vi "serialization tests.vi"() -> (0 "error out":errorcluster, 2 "success?":bool)   [LabVIEW 2013, in "shared memory tests.lvlib"]
doc: "Tests the 'To String' and 'From String' methods of the Module's configuration class and ensures they are compatible."
uses:
  shared memory tests.lvlib
  module/configuration/shared memory configuration.lvclass
  module/configuration/shared memory configuration.lvclass/shared memory configuration.ctl
  <vilib>/NI/Tag Bus Module Framework/channel/TBM channel.lvclass
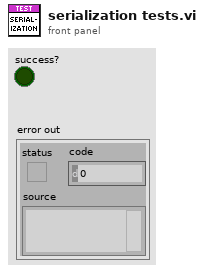
[diagram p1: front panel]
types:
  T1 = typedef "shared memory configuration.lvclass/Line.ctl" = cluster{"channel":refnum<class "TBM channel.lvclass">}
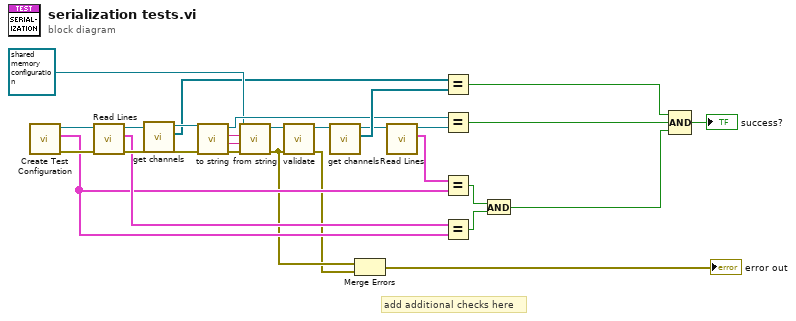
[diagram p0: block diagram]
diagram:
  # "add additional checks here"
  n1 = call "Create Test Configuration.vi"() -> ("error out"=w15:errorcluster, "Line Array"=w10:T1[], "Module Configuration"=w13:refnum<class "shared memory configuration.lvclass">)  [unwired: 6 in, 3 out]
  n2 = call "Read Lines.vi"("error in (no error)"=w15, "shared memory configuration in"=w13) -> ("error out"=w14:errorcluster, "Lines"=w11:T1[], "shared memory configuration out"=w12:refnum<class "shared memory configuration.lvclass">)  [unwired: 7 in]
  n3 = call-dynamic "get channels.vi"("shared memory configuration in"=w12) -> ("channels"=w19:refnum<class "TBM channel.lvclass">[], "shared memory configuration out"=w20:refnum<class "shared memory configuration.lvclass">)  [unwired: 9 in]
  n4 = call-dynamic "to string.vi"("error in"=w14, "shared memory configuration in"=w20) -> ("error out"=w28:errorcluster, "data"=w27:string, "version"=w26:string, "shared memory configuration out"=w22:refnum<class "shared memory configuration.lvclass">)  [unwired: 6 in]
  n5 = call-dynamic "from string.vi"("error in"=w28, "data"=w27, "version"=w26, "shared memory configuration in"=refnum<class "shared memory configuration.lvclass"> refnum ("tag bus configurable plugin module configuration")) -> ("error out"=w7:errorcluster, "shared memory configuration out"=w25:refnum<class "shared memory configuration.lvclass">)  [unwired: 6 in]
  n6 = call-dynamic "validate.vi"("error in"=w7, "shared memory configuration in"=w25) -> ("error out"=w6:errorcluster, "shared memory configuration out"=w24:refnum<class "shared memory configuration.lvclass">)  [unwired: 8 in]
  n7 = call-dynamic "get channels.vi"("shared memory configuration in"=w24) -> ("channels"=w23:refnum<class "TBM channel.lvclass">[], "shared memory configuration out"=w18:refnum<class "shared memory configuration.lvclass">)  [unwired: 9 in]
  n8 = Merge Errors(w7, w6) -> (→"error out":errorcluster)
  n9 = call "Read Lines.vi"("shared memory configuration in"=w18) -> ("Lines"=w16:T1[], "shared memory configuration out"=w17:refnum<class "shared memory configuration.lvclass">)  [unwired: 8 in, 1 out]
  n10 = Equal?(x=w19, y=w23) -> (x = y?=w4:bool)
  n11 = Equal?(x=w22, y=w17) -> (x = y?=w3:bool)
  n12 = Equal?(x=w16, y=w10) -> (x = y?=w9:bool)
  n13 = Equal?(x=w11, y=w10) -> (x = y?=w8:bool)
  n14 = And(x=w9, y=w8) -> (x .and. y?=w2:bool)
  n15 = Compound Arithmetic op=AND(w4, w3, w2) -> (→"success?":bool)
